vi "LSX Set Auto Status.vi"(8 "error in (no error)":errorcluster, 10 "lValue":i32, 11 "lLSID":i32) -> (0 "error out":errorcluster, 3 "function return":i32)   [LabVIEW 2018, in "Tango.lvlib"]
doc: "TANGOAPI int TANGOCALL LSX_SetAutoStatus (int lLSID, int lValue);"
uses:
  <userlib>/Tango/Tango.lvlib
  <userlib>/Tango/Tango_DLL.dll
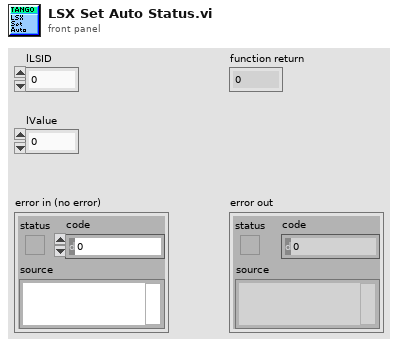
[diagram p1: front panel]
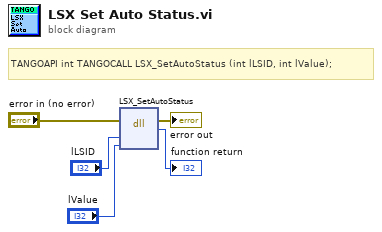
[diagram p0: block diagram]
diagram:
  # "TANGOAPI int TANGOCALL LSX_SetAutoStatus (int lLSID, int lValue);"
  n1 = dll-call lib="C:/Program Files (x86)/National Instruments/LabVIEW 2018/user.lib/Tango/Tango_DLL.*" fn="LSX_SetAutoStatus"(error in="error in (no error)", "lLSID"="lLSID", "lValue"="lValue") -> (error out=→"error out":errorcluster, →"function return":i32)  [unwired: 4 in, 1 out]
